vi "Write INI File.vi"(8 "error in":errorcluster, 11 "Peer Review in":refnum<class "Peer Review.lvclass">) -> (0 "error out":errorcluster, 3 "Peer Review out":refnum<class "Peer Review.lvclass">)   [LabVIEW 2020, in "Peer Review.lvclass"]
uses:
  Peer Review.lvclass
  Peer Review.lvclass/Peer Review.ctl
  <vilib>/Utility/config.llb/Read Key (Path).vi
  <vilib>/Utility/config.llb/Write Key (Path).vi
  <vilib>/Utility/config.llb/Read Key (Boolean).vi
  <vilib>/Utility/config.llb/Write Key (Boolean).vi
  <vilib>/Utility/config.llb/Read Key (String).vi
  <vilib>/Utility/config.llb/Write Key (String).vi
  <vilib>/Utility/config.llb/NI_LVConfig.lvlib
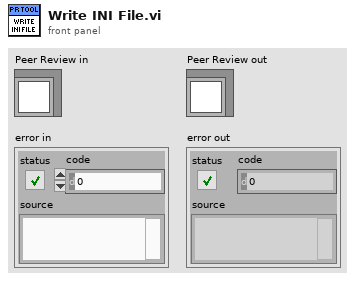
[diagram p1: front panel]
types:
  T1 = typedef "NI_LVConfig.lvlib/Config Data RefNum.ctl" = refnum<k1>
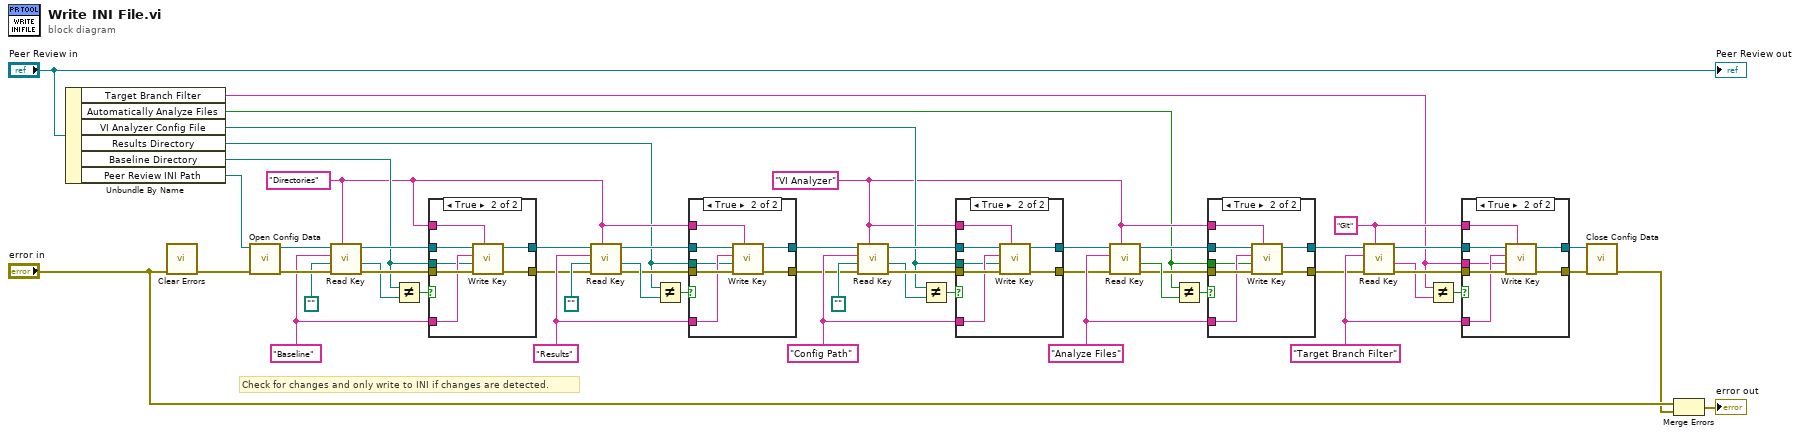
[diagram p0: block diagram]
diagram:
  w4 = "Git" ("section")
  w9 = "Target Branch Filter" ("section")
  w18 = "Analyze Files" ("section")
  w13 = "VI Analyzer" ("section")
  w26 = "Config Path" ("section")
  w37 = "Results" ("section")
  w43 = "Baseline" ("section")
  w31 = "Directories" ("section")
  # "Check for changes and only write to INI if changes are detected."
  n1 = Unbundle By Name("Peer Review in") -> ("Target Branch Filter"=w3:string, "Automatically Analyze Files"=w12:bool, "VI Analyzer Config File"=w21:path, "Results Directory"=w30:path, "Baseline Directory"=w42:path, "Peer Review INI Path"=w49:path)
  n2 = call <vilib>:"Clear Errors.vi"("error in (no error)"="error in") -> ("error out"=w53:errorcluster)  [unwired: 5 in, 1 out]
  n3 = call <vilib>:"Open Config Data.vi"("error in (no error)"=w53, "configuration file path"=w49) -> ("error out"=w45:errorcluster, "refnum"=w48:T1)  [unwired: 7 in, 1 out]
  n4 = call-poly <vilib>:"Read Key.vi"("section"=w31, "error in (no error)"=w45, "default value"=path "", "key"=w43, "refnum"=w48) -> ("error out"=w46:errorcluster, "value"=w41:path, "refnum out"=w47:T1)  [unwired: 3 in, 1 out]
  n5 = Not Equal?(x=w42, y=w41) -> (x != y?=w40:bool)
  n6 = case shown="True" w40 {
    tunnel: [w56 w63] -> w32
    tunnel: [w55 w62] -> w33
    tunnel: w47 -> [w56 w61]
    tunnel: w46 -> [w55 w60]
    tunnel: w31 -> [_ w59]
    tunnel: w43 -> [_ w58]
    tunnel: w42 -> [_ w57]
    frame False {
    }
    frame True {
      n7 = call-poly <vilib>:"Write Key.vi"("section"=w59, "error in (no error)"=w60, "value"=w57, "key"=w58, "refnum"=w61) -> ("error out"=w62:errorcluster, "refnum out"=w63:T1)  [unwired: 4 in, 1 out]
    }
  }
  n8 = call-poly <vilib>:"Read Key.vi"("section"=w31, "error in (no error)"=w33, "default value"=path "", "key"=w37, "refnum"=w32) -> ("error out"=w35:errorcluster, "value"=w38:path, "refnum out"=w34:T1)  [unwired: 3 in, 1 out]
  n9 = Not Equal?(x=w30, y=w38) -> (x != y?=w39:bool)
  n10 = case shown="True" w39 {
    tunnel: [w65 w72] -> w22
    tunnel: [w64 w71] -> w23
    tunnel: w34 -> [w65 w70]
    tunnel: w35 -> [w64 w69]
    tunnel: w31 -> [_ w68]
    tunnel: w37 -> [_ w67]
    tunnel: w30 -> [_ w66]
    frame False {
    }
    frame True {
      n11 = call-poly <vilib>:"Write Key.vi"("section"=w68, "error in (no error)"=w69, "value"=w66, "key"=w67, "refnum"=w70) -> ("error out"=w71:errorcluster, "refnum out"=w72:T1)  [unwired: 4 in, 1 out]
    }
  }
  n12 = call-poly <vilib>:"Read Key.vi"("section"=w13, "error in (no error)"=w23, "default value"=path "", "key"=w26, "refnum"=w22) -> ("error out"=w28:errorcluster, "value"=w25:path, "refnum out"=w29:T1)  [unwired: 3 in, 1 out]
  n13 = Not Equal?(x=w21, y=w25) -> (x != y?=w24:bool)
  n14 = case shown="True" w24 {
    tunnel: [w74 w81] -> w14
    tunnel: [w73 w80] -> w15
    tunnel: w29 -> [w74 w79]
    tunnel: w28 -> [w73 w78]
    tunnel: w13 -> [_ w77]
    tunnel: w26 -> [_ w76]
    tunnel: w21 -> [_ w75]
    frame False {
    }
    frame True {
      n15 = call-poly <vilib>:"Write Key.vi"("section"=w77, "error in (no error)"=w78, "value"=w75, "key"=w76, "refnum"=w79) -> ("error out"=w80:errorcluster, "refnum out"=w81:T1)  [unwired: 4 in, 1 out]
    }
  }
  n16 = call-poly <vilib>:"Read Key.vi"("section"=w13, "error in (no error)"=w15, "key"=w18, "refnum"=w14) -> ("error out"=w17:errorcluster, "value"=w19:bool, "refnum out"=w16:T1)  [unwired: 4 in, 1 out]
  n17 = Not Equal?(x=w12, y=w19) -> (x != y?=w20:bool)
  n18 = case shown="True" w20 {
    tunnel: [w83 w90] -> w6
    tunnel: [w82 w89] -> w5
    tunnel: w16 -> [w83 w88]
    tunnel: w17 -> [w82 w87]
    tunnel: w13 -> [_ w86]
    tunnel: w18 -> [_ w85]
    tunnel: w12 -> [_ w84]
    frame False {
    }
    frame True {
      n19 = call-poly <vilib>:"Write Key.vi"("section"=w86, "error in (no error)"=w87, "value"=w84, "key"=w85, "refnum"=w88) -> ("error out"=w89:errorcluster, "refnum out"=w90:T1)  [unwired: 4 in, 1 out]
    }
  }
  n20 = call-poly <vilib>:"Read Key.vi"("section"=w4, "error in (no error)"=w5, "key"=w9, "refnum"=w6) -> ("error out"=w10:errorcluster, "value"=w8:string, "refnum out"=w11:T1)  [unwired: 4 in, 1 out]
  n21 = Not Equal?(x=w3, y=w8) -> (x != y?=w7:bool)
  n22 = case shown="True" w7 {
    tunnel: [w92 w99] -> w2
    tunnel: [w91 w98] -> w1
    tunnel: w11 -> [w92 w97]
    tunnel: w10 -> [w91 w96]
    tunnel: w4 -> [_ w95]
    tunnel: w9 -> [_ w94]
    tunnel: w3 -> [_ w93]
    frame False {
    }
    frame True {
      n23 = call-poly <vilib>:"Write Key.vi"("section"=w95, "error in (no error)"=w96, "value"=w93, "key"=w94, "refnum"=w97) -> ("error out"=w98:errorcluster, "refnum out"=w99:T1)  [unwired: 4 in, 1 out]
    }
  }
  n24 = call <vilib>:"Close Config Data.vi"("error in (no error)"=w1, "refnum"=w2) -> ("error out"=w52:errorcluster)  [unwired: 8 in, 1 out]
  n25 = Merge Errors("error in", w52) -> (→"error out":errorcluster)
  "Peer Review out" <- "Peer Review in"
